vi "UDP.Rx.Top.vi"(8 "error in (no error)":errorcluster, 9 "max size (800)":i32=800, 10 "ports":u16[](array[numeric])=[60000, 60001, 60002, 60003], 11 "Stop Pointer":refnum<class "Memory.Pointer.lvclass">) -> (0 "error out":errorcluster)   [LabVIEW 2017]
uses:
  <vilib>/NI/Memory Manager/Classes/Pointer/Memory.Pointer.lvclass
  <vilib>/NI/Memory Manager/Classes/Pointer/Memory.Pointer.lvclass/Memory.Pointer.ctl
  <vilib>/NI/Memory Manager/Classes/Pointer/Memory.Pointer.Read.0D.I32.vi
  <vilib>/NI/Memory Manager/Classes/Pointer/Memory.Pointer.Write.0D.Bool.vi
  <vilib>/NI/Memory Manager/Classes/Pointer/Memory.Pointer.Read.0D.Bool.vi
  <vilib>/NI/Memory Manager/Classes/Pointer/Memory.Pointer.Read.No Check.0D.I32.vi
  <vilib>/NI/Memory Manager/Classes/Pointer/Memory.Pointer.Parameter Check.Null Pointer.vi
  <vilib>/NI/Memory Manager/Classes/Pointer/Memory.Pointer.Parameter Check.Subset.vi
  <vilib>/NI/Memory Manager/Classes/Pointer/Memory.Pointer.Write.No Check.0D.Bool.vi
  <vilib>/NI/Memory Manager/Classes/Pointer/Memory.Pointer.Read.No Check.0D.Bool.vi
  <vilib>/NI/Memory Manager/Classes/Pointer/Memory.Pointer.Get Address.vi
  <vilib>/NI/Memory Manager/Classes/Pointer/Memory.Pointer.Errors.vi
  <vilib>/NI/Memory Manager/Classes/Pointer/Memory.Pointer.Errors.Null Pointer.vi
  <vilib>/NI/Memory Manager/Classes/Pointer/Memory.Pointer.Errors.Out of Bounds.vi
  <vilib>/NI/Memory Manager/Classes/Pointer/Memory.Pointer.Get Size.vi
  <vilib>/NI/Memory Manager/Classes/Pointer/Memory.Pointer.Errors.Create Error.vi
  <vilib>/NI/Memory Manager/VIs/Source.Write.String.vi
  <vilib>/NI/Memory Manager/Classes/Pointer/Memory.Pointer.Errors.Write Pointer Size.vi
  <vilib>/NI/Memory Manager/VIs/Source.Write.Scalar.Base10.vi
  <vilib>/NI/Memory Manager/VIs/Source.Write.Scalar.Base10 (U64).vi
  <vilib>/NI/Memory Manager/VIs/New Error Cluster Constant.vi
  <vilib>/NI/Memory Manager/VIs/New Error Cluster Constant (512B).vi
  <vilib>/NI/Memory Manager/VIs/Error Cluster.Set Status.vi
  <vilib>/NI/Memory Manager/VIs/Error Cluster.Set Code.vi
  <vilib>/NI/Memory Manager/VIs/Error Cluster.Set VI Source.vi
  <vilib>/NI/Memory Manager/Constants/Memory.Constants.vi
  <vilib>/NI/Memory Manager/Constants/Memory.Constants.Library Name.vi
  <vilib>/NI/Memory Manager/Classes/Pointer/Memory.Pointer.Errors.Get Info.vi
panel:
  out "rx counts":i32[](array[numeric])
  in  "Stop":bool
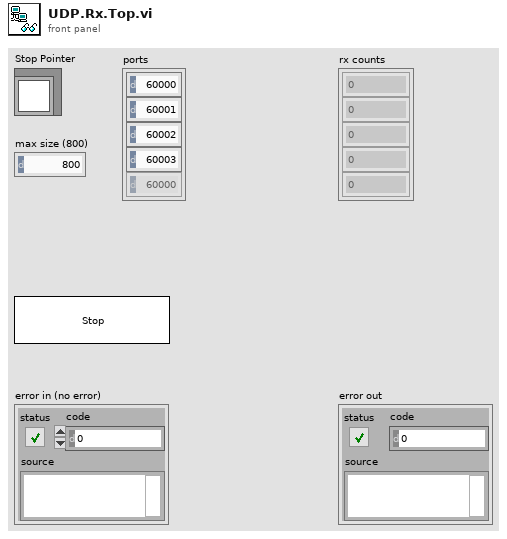
[diagram p1: front panel]
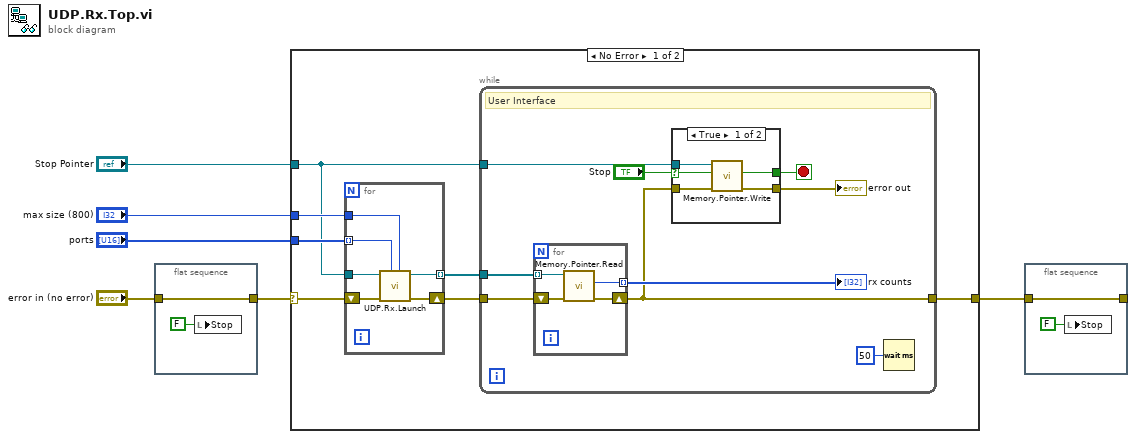
[diagram p0: block diagram]
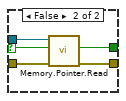
[diagram p2: hidden frame]
diagram:
  n1 = flat-sequence {
    tunnel: "error in (no error)" -> [w8]
    tunnel: [w8] -> w1
    frame #0 {
      n2 = local write "Stop"(FALSE ("Stop")) -> ()
    }
  }
  n3 = case shown="No Error" w1 {
    selector: w1 -> [w9 w45]
    tunnel: "ports" -> [w15 _]
    tunnel: "max size (800)" -> [w14 _]
    tunnel: "Stop Pointer" -> [w11 _]
    tunnel: [w10 w45] -> w2
    frame No Error {
      n4 = for {
        tunnel: w11 -> [w16]
        tunnel: w15 -> [w19] mode=indexing
        tunnel: w14 -> [w18]
        shift-right: [w21] -> w13
        shift-left: w9 -> [w20]
        tunnel: [w17] -> w12 mode=indexing
        n5 = call "UDP.Rx.Launch.vi"("max size (548)"=w18, "port"=w19, "error in (no error)"=w20, "Stop Pointer"=w16) -> ("error out"=w21:errorcluster, "Count Pointer"=w17:refnum<class "Memory.Pointer.lvclass">)  [unwired: 6 in]
      }
      n6 = while {
        tunnel: w13 -> [w29]
        tunnel: w12 -> [w30]
        tunnel: w11 -> [w28]
        tunnel: [w22] -> w10
        stop <- w27 stop-if-true
        # "User Interface"
        n7 = for {
          tunnel: w30 -> [w44] mode=indexing
          tunnel: [w42] -> w24 mode=indexing
          shift-right: [w41] -> w22
          shift-left: w29 -> [w43]
          n8 = call-poly <vilib>:"Memory.Pointer.Read.vi"("error in (no error)"=w43, "Pointer in"=w44) -> ("error out"=w41:errorcluster, "value out"=w42:i32)  [unwired: 6 in, 2 out]
        }
        "rx counts" <- w24
        n9 = case shown="True" "Stop" {
          selector: "Stop" -> [w31 w36]
          tunnel: w28 -> [w35 w40]
          tunnel: w22 -> [w34 w39]
          tunnel: [w33 w38] -> w27
          tunnel: [w32 w37] -> w25
          frame True {
            n10 = call-poly <vilib>:"Memory.Pointer.Write.vi"("error in (no error)"=w34, "value"=w31, "Pointer in"=w35) -> ("error out"=w32:errorcluster, "value"=w33:bool)  [unwired: 5 in, 2 out]
          }
          frame False {
            n11 = call-poly <vilib>:"Memory.Pointer.Read.vi"("error in (no error)"=w39, "value in"=w36, "Pointer in"=w40) -> ("error out"=w37:errorcluster, "value out"=w38:bool)  [unwired: 5 in, 2 out]
          }
        }
        "error out" <- w25
        n12 = Wait (ms)(milliseconds to wait=u32 50) -> ()  [unwired: 1 out]
      }
    }
    frame Error {
    }
  }
  n13 = flat-sequence {
    tunnel: w2 -> [w47]
    tunnel: [w47] -> _
    frame #0 {
      n14 = local write "Stop"(FALSE ("Stop")) -> ()
    }
  }
